vi "Configure Custom Auto-Averaging.vi"(0 "reference":refnum<k15>, 5 "Initial Aperture Time (s)":dbl=0.00025 format="%#_13p", 11 "error in (no error)":errorcluster) -> (4 "reference out":refnum<k15>, 15 "error out":errorcluster)   [LabVIEW 2023, in "NI-568x RF Power Meter.lvlib" / "SG 2250 Path Accessor.lvclass"]
uses:
  SG 2250 Path Accessor.lvclass
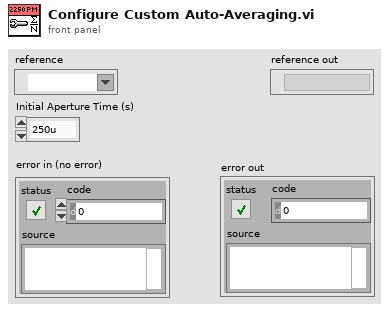
[diagram p1: front panel]
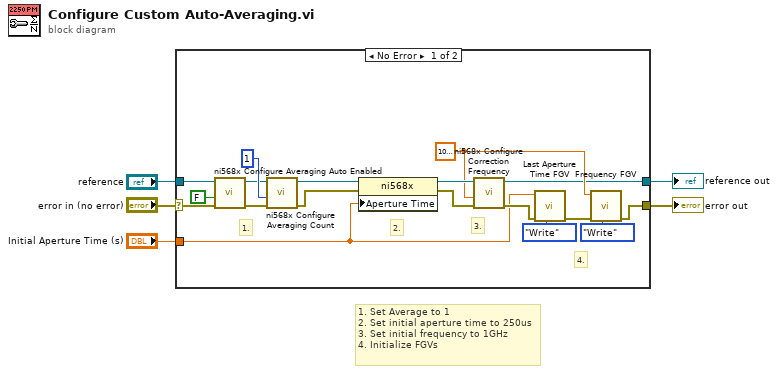
[diagram p0: block diagram]
diagram:
  # "1. Set Average to 1\n2. Set initial aperture time to 250us\n3. Set initial frequency to 1GHz\n4. Initialize FGVs"
  n1 = case shown="No Error" "error in (no error)" {
    selector: "error in (no error)" -> [w12 w25]
    tunnel: [w14 w24] -> w3
    tunnel: [w21 w25] -> w5
    tunnel: "reference" -> [w13 w24]
    tunnel: "Initial Aperture Time (s)" -> [w6 _]
    frame No Error {
      w15 = 1000000000.0 ("Write Value (Hz)")
      # "4."
      # "3."
      # "2."
      # "1."
      n2 = call <instrlib>:"ni568x Configure Averaging Auto Enabled.vi"("error in"=w12, "auto averaging enabled"=FALSE, "instrument handle"=w13) -> ("error out"=w11:errorcluster, "instrument handle out"=w18:refnum<k15>)  [unwired: 7 in]
      n3 = call <instrlib>:"ni568x Configure Averaging Count.vi"("error in"=w11, "averaging count"=u32 1 ("NbrAverages"), "instrument handle"=w18) -> ("error out"=w10:errorcluster, "instrument handle out"=w17:refnum<k15>)  [unwired: 7 in]
      n4 = property class="ni568x"(reference=w17, error in=w10, "Aperture Time"=w6) -> (reference out=w16:refnum<k15>, error out=w9:errorcluster)
      n5 = call <instrlib>:"ni568x Configure Correction Frequency.vi"("error in"=w9, "frequency"=w15, "instrument handle"=w16) -> ("error out"=w8:errorcluster, "instrument handle out"=w14:refnum<k15>)  [unwired: 7 in]
      n6 = call "Last Aperture Time FGV.vi"("Action"=enum16{"Write", "Read"}."Write", "error in (no error)"=w8, "Write Value (s)"=w6) -> ("error out"=w22:errorcluster)  [unwired: 4 in, 1 out]
      n7 = call "Frequency FGV.vi"("Action"=enum16{"Write", "Read"}."Write", "error in (no error)"=w22, "Write Value (Hz)"=w15) -> ("error out"=w21:errorcluster)  [unwired: 4 in, 1 out]
    }
    frame Error {
    }
  }
  "error out" <- w5
  "reference out" <- w3
